vi "Write and Read Multiple Holding Registers.vi"(4 "read count":u16, 6 "read operation starting address":u16, 8 "error in (no error)":errorcluster, 9 "values to write":u16[](array[numeric]), 10 "write operation starting address":u16, 11 "Modbus master in":refnum<class "Modbus Master.lvclass">) -> (0 "error out":errorcluster, 1 "values read":u16[](array[numeric]), 3 "Modbus master out":refnum<class "Modbus Master.lvclass">)   [LabVIEW 2021, in "Modbus Master.lvclass"]
doc: "Writes and reads values to and from contiguous holding registers. This VI performs the write operation before the read operation. The maximum number of holding registers this VI can write is 121. The maximum number of holding registers this VI can read is 125."
uses:
  Modbus Master.lvclass
  Modbus Master.lvclass/Modbus Master.ctl
  Modbus Data Unit/Modbus Data Unit.lvclass/Modbus Data Unit.ctl
  Network Protocol/Network Master/Network Master.lvclass/Network Master.ctl
  Master Function Definition/Write and Read Multiple Registers Request.vi
  Master Function Definition/Function data mismatch error.vi
  Master Function Definition/Write and Read Multiple Registers Response.vi
  Network Protocol/Network Master/Read write Master.vi
  Modbus Data Unit/Construct PDU.vi
  Utility/U16s to Bytes.vi
  Utility/Bytes to U16s.vi
  Master Function Definition/Function code mismatch error.vi
  Data Model/Error Generator.vi
  Modbus Data Unit/Deconstruct PDU.vi
  Modbus Data Unit/Modbus Data Unit.lvclass
  Transmission Data Unit/Transmission Data Unit.lvclass
  Network Protocol/Network Master/Network Master.lvclass
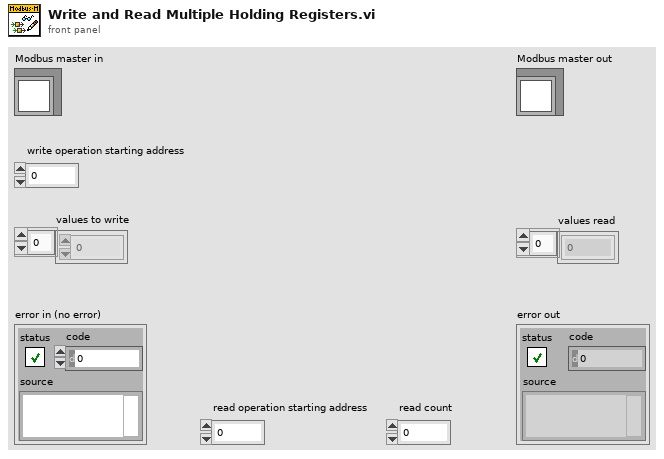
[diagram p1: front panel]
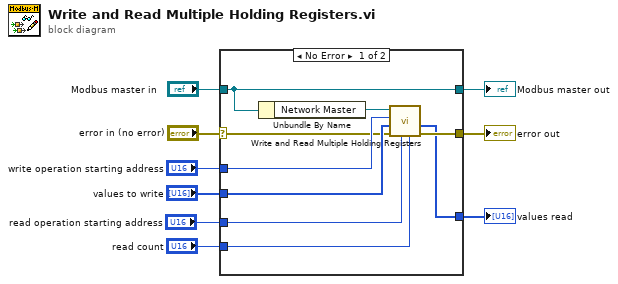
[diagram p0: block diagram]
diagram:
  n1 = case shown="No Error" "error in (no error)" {
    selector: "error in (no error)" -> [w11 w19]
    tunnel: "Modbus master in" -> [w10 w20]
    tunnel: [w10 w20] -> w8
    tunnel: [w18 w19] -> w7
    tunnel: "read count" -> [w14 _]
    tunnel: [w13 _] -> w4
    tunnel: "read operation starting address" -> [w15 _]
    tunnel: "values to write" -> [w17 _]
    tunnel: "write operation starting address" -> [w16 _]
    frame No Error {
      n2 = Unbundle By Name(w10) -> ("Network Master"=w12:refnum<class "Network Master.lvclass">)
      n3 = call "Write and Read Multiple Holding Registers.vi"("read count"=w14, "read operation starting address"=w15, "error in (no error)"=w11, "values to write"=w17, "write operation starting address"=w16, "Modbus master in"=w12) -> ("error out"=w18:errorcluster, "values read"=w13:u16[])  [unwired: 3 in, 1 out]
    }
    frame Error {
    }
  }
  "error out" <- w7
  "Modbus master out" <- w8
  "values read" <- w4
